vi "UI_Loop_Error_Queue_Setup.vi"(8 "error in":errorcluster) -> (0 "error out":errorcluster, 5 "queue out":refnum<queue>)   [LabVIEW 2021]
uses:
  Controles/Main_Machine_State.ctl
  Controles/Command(ERD Loop Control).ctl
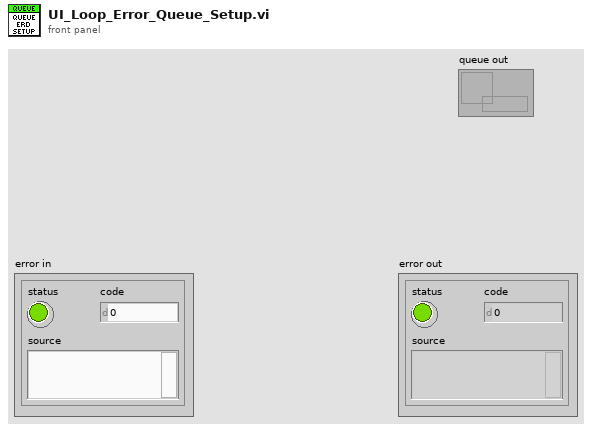
[diagram p1: front panel]
types:
  T1 = typedef "Command(ERD Loop Control).ctl" = enum16{"Initialize", "Shutdown"}
  T2 = typedef "Main_Machine_State.ctl" = enum16{"Init", "Get Version", "Build ERD Read List", "Update UI", "Read ERDs", "Log Data", "Pause", "Shutdown"}
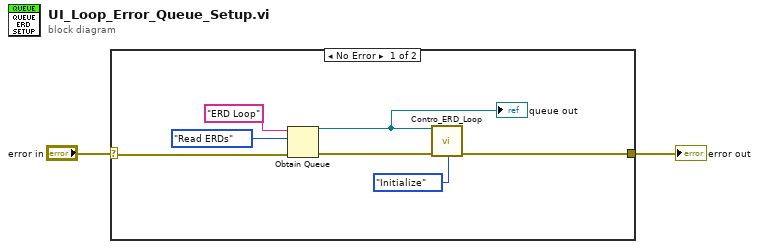
[diagram p0: block diagram]
diagram:
  n1 = case shown="No Error" "error in" {
    selector: "error in" -> [w4 w10]
    tunnel: [w3 w10] -> w1
    frame No Error {
      n2 = Obtain Queue(name (unnamed)="ERD Loop", element data type=Main_Machine_State."Read ERDs", error in (no error)=w4) -> (queue out=w6:refnum<queue>, error out=w7:errorcluster)  [unwired: 2 in, 1 out]
      "queue out" <- w6
      n3 = call "Contro_ERD_Loop.vi"("ERD Loop"=w6, "Error In"=w7, "Command (ERD Loop Control)"=Command(ERD_Loop_Control)."Initialize") -> ("Error Out"=w3:errorcluster)  [unwired: 12 in]
    }
    frame Error {
    }
  }
  "error out" <- w1
